vi "PythonPDF.vi"(5 "data_values":string[](array[string])=["March 16, 2022", "123", "1234", "Tristan Lee", "5kw", "VI test", "12345", "P", "P", "P", "P", "P", "54.00", "0.1", "P", "P", "P", "P", "58.01", "48.00", "54.08", "-0.5", "-0.1", "0", "52.0", "45.0", "=F36*F35", "50.0", "26", "P"], 7 "data_names":string[](array[string])=["$!Test_Date", "$!Part_No", "$!Serial_No", "$!Tested_By", "$!station_ID", "$!Comments", "$!FW_Rev", "$!6.1.", "$!6.2.", "$!6.3.", "$!6.4.3.", "$!6.4.4.", "$!6.4.5.", "$!6.5.5.", "$!6.6.3.", "$!6.6.4.", "$!6.6.5.", "$!6.6.6.", "$!6.7.2.", "$!6.7.4.", "$!6.7.5.", "$!6.8.3.", "$!6.8.4.", "$!6.8.5.", "$!6.9.1.", "$!6.9.2.", "$!6.9.3.", "$!6.9.6.", "$!6.9.10.", "$!6.10."], 8 "pdf_path":string="C:\\Users\\trist\\Desktop\\Desktop\\UBC Engineering\\Coop\\Alpha\\Work\\Python\\PyLab_PDF proj\\templates\\results.pdf", 9 "results_path":path=path "C:/Users/trist/Desktop/Desktop/UBC Engineering/Coop/Alpha/Work/Python/PyLab_PDF proj/templates/results.xlsx", 10 "tempalte_path":path=path "C:/Users/trist/Desktop/Desktop/UBC Engineering/Coop/Alpha/Work/Python/PyLab_PDF proj/templates/0100048-A5_R_1.xltx", 11 "module path":path=path "C:/Users/trist/Desktop/Desktop/UBC Engineering/Coop/Alpha/Work/Python/PyLab_PDF proj/PythonPDF.py") -> ()   [LabVIEW 2020]
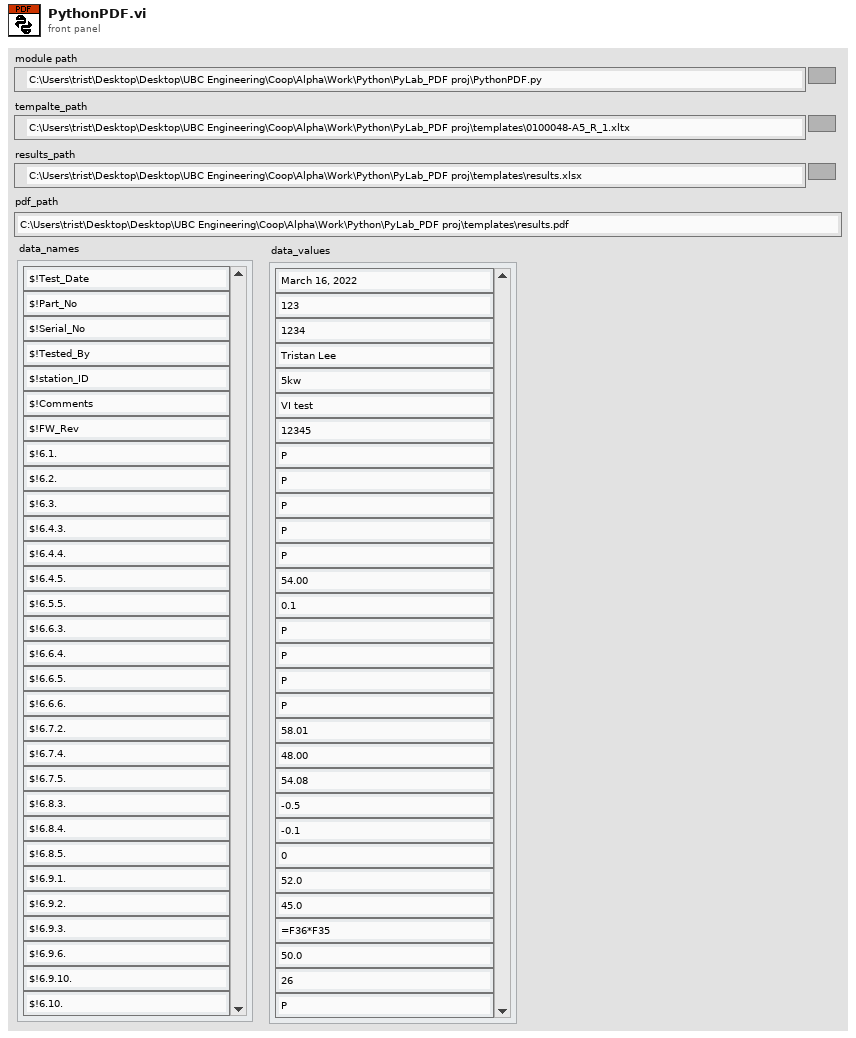
[diagram p1: front panel]
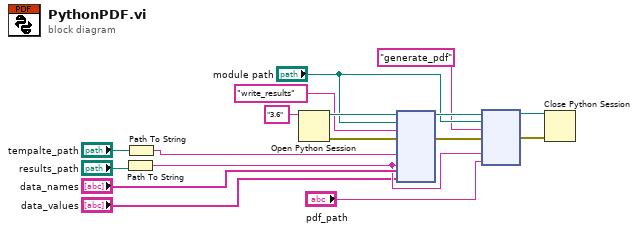
[diagram p0: block diagram]
diagram:
  n1 = Path To String(path="results_path") -> (string=w2:string)
  n2 = Path To String(path="tempalte_path") -> (string=w3:string)
  n3 = Open Python Session(python version="3.6" ("Python version")) -> (session out=w17:refnum<k35>, error out=w16:errorcluster)  [unwired: 2 in]
  n4 = node(w17, "module path", "write_results", w16, w3, w2, "data_names", "data_values") -> (w13:refnum<k35>, w12:errorcluster)  [unwired: 6 in, 2 out]
  n5 = node(w13, "module path", "generate_pdf" ("function name"), w12, w2, "pdf_path") -> (w7:refnum<k35>, w6:errorcluster)  [unwired: 4 in, 2 out]
  n6 = Close Python Session(session in=w7, error in=w6) -> ()  [unwired: 1 out]
